vi "Working Thread.vi"(7 "EngineCSM":string, 10 "SocketName":string, 11 "Sequence":string) -> ()   [LabVIEW 2020, in "CSMStand(Lite).lvlib"]
uses:
  CSMStand(Lite).lvlib
  Typedef/Def-StepComplete Event Data.ctl
  162d78b0-f25f-4e28-9f32-62a227129c30.vi
  3235fbb5-1003-4f8d-8a8e-733f49405df1.vi
  29c90474-5633-4ebd-9475-c7049fde7730.vi
  07558781-58e1-4dd2-b95a-dcbf6018b6a4.vi
  <userlib>/_NEVSTOP/Communicable State Machine(CSM)/AdvanceAPI/CSM - Set Module Attribute.vi
  <userlib>/_NEVSTOP/Communicable State Machine(CSM)/addons/API-String-Arugments-Support/_Support/Data To API String Arguments.vi
  <userlib>/_NEVSTOP/Communicable State Machine(CSM)/AdvanceAPI/CSM - Get Module Attribute.vi
  <userlib>/_NEVSTOP/Communicable State Machine(CSM)/Communicable State Machine.lvlib
  <userlib>/_NEVSTOP/Communicable State Machine(CSM)/_Shared/CSM Shared.lvlib
  <userlib>/_NEVSTOP/Communicable State Machine(CSM)/addons/API-String-Arugments-Support/API String Arguments Support.lvlib
panel:
  in  "Debug Stop":bool
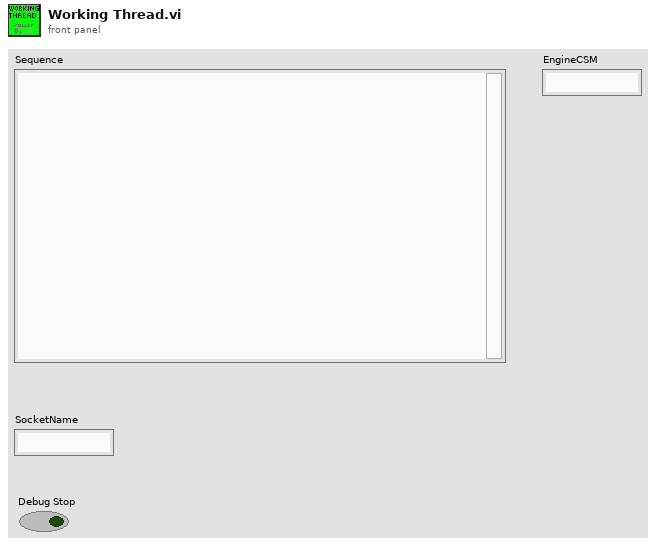
[diagram p1: front panel]
types:
  T1 = typedef "CSMStand(Lite).lvlib/Def-StepComplete Event Data.ctl" = cluster{"index":i32, "Arguments":string, "error":errorcluster}
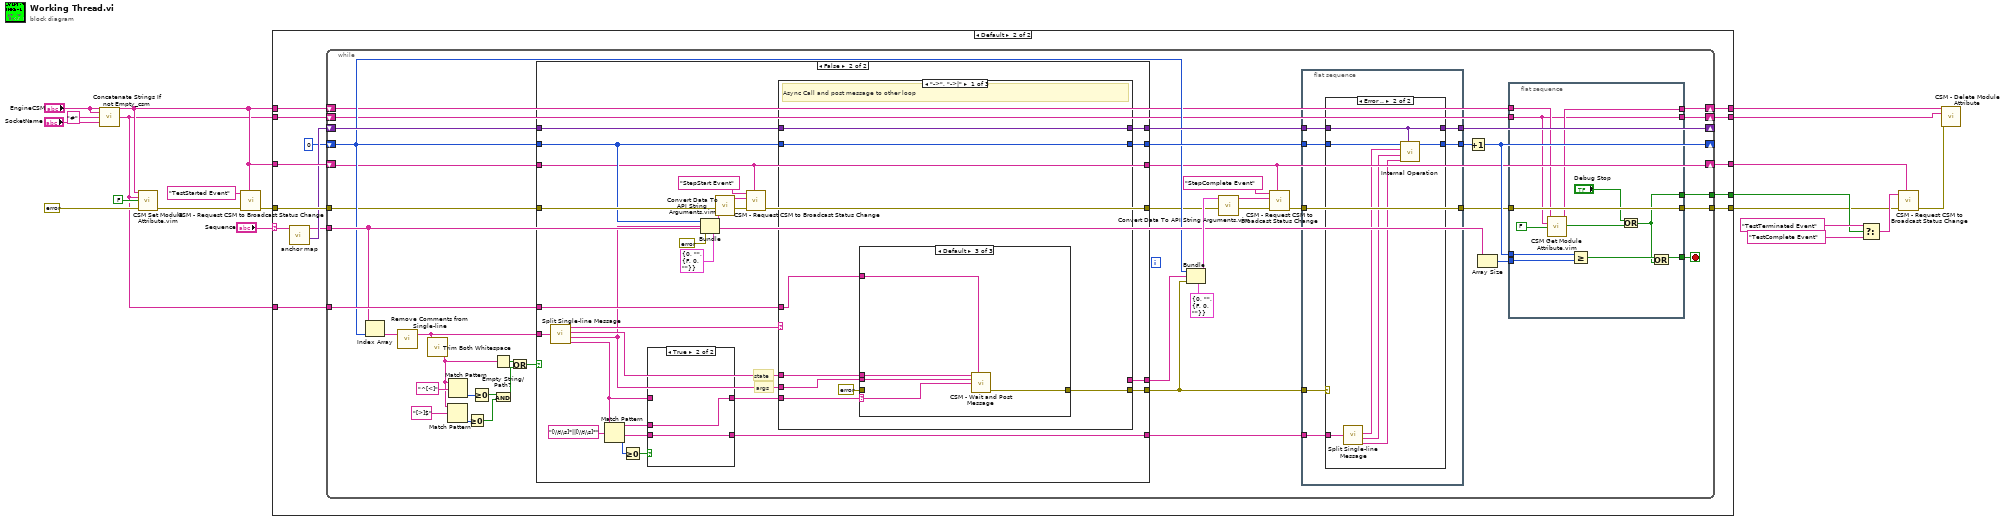
[diagram p0: block diagram]
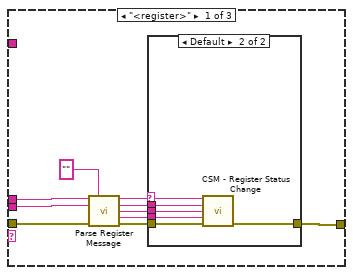
[diagram p6: hidden frame]
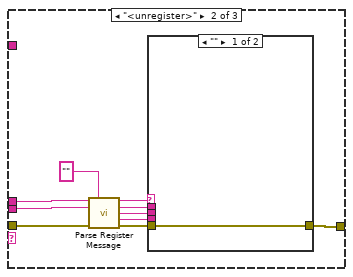
[diagram p8: hidden frame]
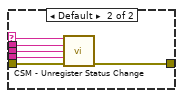
[diagram p9: hidden frame]
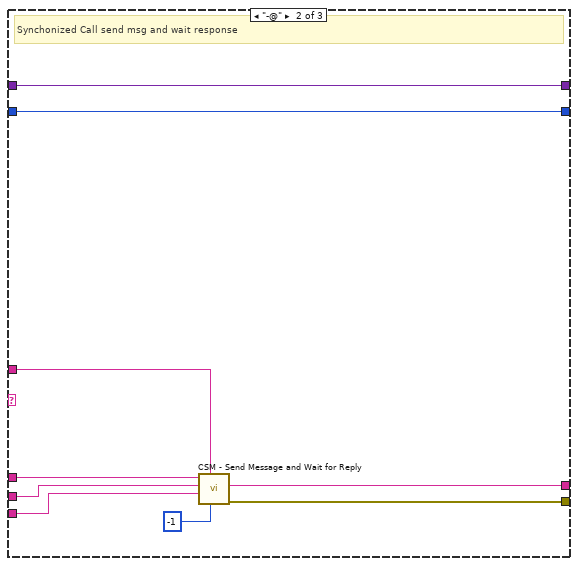
[diagram p10: hidden frame]
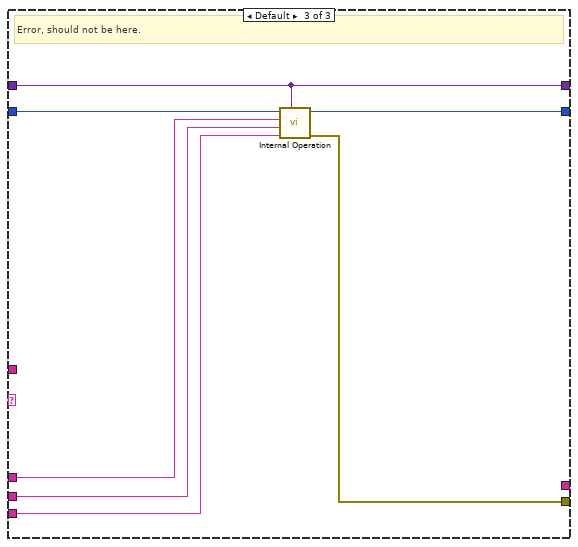
[diagram p11: hidden frame]
diagram:
  n1 = call <userlib>:"Concatenate Strings If not Empty_csm.vi"("String"="SocketName", "seperator(:)"="#", "prefix"="EngineCSM") -> ("result"=w1:string)  [unwired: 2 in]
  n2 = call "CSM Set Module Attribute.vim"("CSM Name"="EngineCSM", "Attribute"=w1, "Value"=FALSE, "Error In"=errorcluster {"status"=FALSE, "code"=0, "source"=""} ("error in (no error)")) -> ("error out"=w5:errorcluster)  [unwired: 8 in, 3 out]
  n3 = call <userlib>:"CSM - Request CSM to Broadcast Status Change.vi"("Module Name"="EngineCSM", "Error In (No Error)"=w5, "Status"="TestStarted Event") -> ("error out"=w18:errorcluster)  [unwired: 8 in]
  n4 = case shown="Default" "Sequence" {
    selector: "Sequence" -> [_ w31]
    tunnel: w18 -> [w22 w37]
    tunnel: "EngineCSM" -> [w23 w36]
    tunnel: [w23 w35] -> w17
    tunnel: [w22 w34] -> w9
    tunnel: w1 -> [_ w33]
    tunnel: "EngineCSM" -> [w21 w28]
    tunnel: [w21 w27] -> w12
    tunnel: [_ w26] -> w10
    tunnel: w1 -> [w20 w25]
    tunnel: [w20 w24] -> w6
    frame "False" {
    }
    frame Default {
      n5 = call "anchor map.vi"("string"=w31) -> ("Archt Map"=w32:variant, "Lines"=w30:string[])  [unwired: 9 in]
      n6 = while {
        tunnel: w37 -> [w43]
        tunnel: [w73] -> w34
        shift-right: [w40] -> w35
        shift-left: w36 -> [w41]
        tunnel: w33 -> [w80]
        tunnel: w30 -> [w70]
        shift-right: [w71] -> _
        shift-left: 0 -> [w47]
        shift-right: [w61] -> _
        shift-left: w32 -> [w68]
        shift-right: [w45] -> w27
        shift-left: w28 -> [w46]
        tunnel: [w44] -> w26
        shift-right: [w38] -> w24
        shift-left: w25 -> [w39]
        stop <- w74 stop-if-true
        n7 = Index Array(array=w70, index=w47) -> (element=w72:string)
        n8 = call <userlib>:"Remove Comments from Single-line.vi"("single-line text"=w72) -> ("single-line text without comments"=w52:string)  [unwired: 2 in]
        n9 = call <userlib>:"Trim Both Whitespace.vi"("String"=w52) -> ("Trimmed String"=w51:string)  [unwired: 1 in]
        n10 = Match Pattern(string=w51, regular expression="[>]$") -> (offset past match=w57:i32)  [unwired: 1 in, 3 out]
        n11 = Match Pattern(string=w51, regular expression="^[<]") -> (offset past match=w58:i32)  [unwired: 1 in, 3 out]
        n12 = Greater Or Equal To 0?(x=w57) -> (x >= 0?=w56:bool)
        n13 = Greater Or Equal To 0?(x=w58) -> (x >= 0?=w55:bool)
        n14 = Empty String/Path?(string/path=w51) -> (empty?=w53:bool)
        n15 = And(x=w55, y=w56) -> (x .and. y?=w54:bool)
        n16 = Or(x=w53, y=w54) -> (x .or. y?=w50:bool)
        n17 = case shown="False" w50 {
          tunnel: w80 -> [_ w138]
          tunnel: [_ w137] -> w64
          tunnel: [_ w136] -> w76
          tunnel: [w112 w135] -> w48
          tunnel: w47 -> [w112 w115]
          tunnel: w68 -> [w111 w134]
          tunnel: [_ w126] -> w63
          tunnel: [w111 w125] -> w62
          tunnel: w52 -> [_ w124]
          tunnel: w43 -> [w110 w120]
          tunnel: [w110 w119] -> w42
          tunnel: w41 -> [w109 w113]
          tunnel: [w109 w113] -> w40
          frame True {
          }
          frame False {
            # "args"
            # "state"
            n18 = call <userlib>:"Split Single-line Message.vi"("single-line text"=w124) -> ("operator"=w140:string, "state"=w139:string, "args"=w114:string, "source/target"=w129:string)  [unwired: 6 in]
            n19 = Match Pattern(string=w129, regular expression="[\\t\\s]*||[\\t\\s]*" ("string")) -> (before substring=w132:string, after substring=w127:string, offset past match=w131:i32)  [unwired: 1 in, 1 out]
            n20 = Greater Or Equal To 0?(x=w131) -> (x >= 0?=w130:bool)
            n21 = case shown="True" w130 {
              tunnel: w132 -> [_ w143]
              tunnel: w129 -> [w141 _]
              tunnel: [w141 w143] -> w128
              tunnel: w127 -> [_ w142]
              tunnel: [_ w142] -> w126
              frame False {
              }
              frame True {
              }
            }
            n22 = Bundle(cluster=T1 {"index"=0, "Arguments"="", "error"={"status"=FALSE, "code"=0, "source"=""}} ("output cluster"), "index"=w115, "Arguments"=w114, "error"=errorcluster {"status"=FALSE, "code"=0, "source"=""}) -> (w117:T1)
            n23 = call "Convert Data To API String Arguments.vim"("error in (no error)"=w120, "data"=w117) -> ("error out"=w122:errorcluster, "String"=w121:string)  [unwired: 6 in]
            n24 = call <userlib>:"CSM - Request CSM to Broadcast Status Change.vi"("Module Name"=w113, "Error In (No Error)"=w122, "Arguments (\"\")"=w121, "Status"="StepStart Event") -> ("error out"=w119:errorcluster)  [unwired: 7 in]
            n25 = case shown="\"->\", \"->|\"" w140 {
              tunnel: w139 -> [w147 w196 w201]
              tunnel: w114 -> [w146 w195 w200]
              tunnel: w138 -> [w148 w197 _]
              tunnel: w128 -> [w145 w194 w199]
              tunnel: [w149 w192 w202] -> w137
              tunnel: [_ w191 _] -> w136
              tunnel: [w151 w190 w204] -> w135
              tunnel: w115 -> [w151 w190 w203]
              tunnel: w134 -> [w150 w189 w198]
              tunnel: [w150 w189 w198] -> w125
              frame "->", "->|" {
                # "Async Call and post message to other loop"
                n26 = case shown="Default" w145 {
                  selector: w145 -> [_ _ w188]
                  tunnel: w146 -> [w155 w171 w187]
                  tunnel: w147 -> [w156 w172 w186]
                  tunnel: errorcluster {"status"=FALSE, "code"=0, "source"=""} ("error IO") -> [w154 w170 _]
                  tunnel: [w153 w169 w184] -> w149
                  tunnel: w148 -> [_ _ w185]
                  frame "<register>" {
                    n27 = call <userlib>:"Parse Register Message.vi"("State"=w156, "Module Name"="", "Args"=w155) -> ("Target"=w160:string, "Source"=w159:string, "Status"=w158:string, "Api"=w157:string)  [unwired: 8 in, 1 out]
                    n28 = case shown="Default" w160 {
                      selector: w160 -> [_ w167]
                      tunnel: w159 -> [_ w166]
                      tunnel: w158 -> [_ w165]
                      tunnel: w157 -> [_ w164]
                      tunnel: w154 -> [w161 w163]
                      tunnel: [w161 w162] -> w153
                      frame "" {
                      }
                      frame Default {
                        n29 = call <userlib>:"CSM - Register Status Change.vi"("CSM Name"=w167, "Source CSM Name (* as Default)"=w166, "Status"=w165, "Response Message (If \"\", Same as Source Message)"=w164, "Error In"=w163) -> ("error out"=w162:errorcluster)  [unwired: 9 in, 1 out]
                      }
                    }
                  }
                  frame "<unregister>" {
                    n30 = call <userlib>:"Parse Register Message.vi"("State"=w172, "Module Name"="", "Args"=w171) -> ("Target"=w176:string, "Source"=w175:string, "Status"=w174:string, "Api"=w173:string)  [unwired: 8 in, 1 out]
                    n31 = case shown="\"\"" w176 {
                      selector: w176 -> [_ w183]
                      tunnel: w175 -> [_ w182]
                      tunnel: w174 -> [_ w181]
                      tunnel: w173 -> [_ w180]
                      tunnel: w170 -> [w177 w179]
                      tunnel: [w177 w178] -> w169
                      frame "" {
                      }
                      frame Default {
                        n32 = call <userlib>:"CSM - Unregister Status Change.vi"("CSM Name"=w183, "Source CSM Name (* as Default)"=w182, "Status"=w181, "Response Message (\"*\" as Default)"=w180, "Error In"=w179) -> ("error out"=w178:errorcluster)  [unwired: 9 in, 1 out]
                      }
                    }
                  }
                  frame Default {
                    n33 = call <userlib>:"CSM - Wait and Post Message.vi"("State"=w186, "Current Module (\"\" to Generate an ID)"=w185, "Arguments (\"\")"=w187, "Target Module"=w188) -> ("error out"=w184:errorcluster)  [unwired: 11 in]
                  }
                }
              }
              frame "-@" {
                # "Synchonized Call send msg and wait response"
                n34 = call <userlib>:"CSM - Send Message and Wait for Reply.vi"("Response Timeout (-2 Using Global Settings)"=-1 ("Response Timeout(5000ms)"), "Current Module (\"\" to Generate an ID)"=w197, "Target Module"=w194, "Arguments (\"\")"=w195, "State"=w196) -> ("error out"=w192:errorcluster, "Response"=w191:string)  [unwired: 4 in, 1 out]
              }
              frame Default {
                # "Error, should not be here."
                n35 = call "Internal Operation.vi"("Archt Map"=w198, "source/target"=w199, "args"=w200, "state"=w201, "Numeric in"=w203) -> ("error out"=w202:errorcluster, "Numeric out"=w204:i32)  [unwired: 5 in]
              }
            }
          }
        }
        n36 = Bundle(cluster=T1 {"index"=0, "Arguments"="", "error"={"status"=FALSE, "code"=0, "source"=""}} ("output cluster"), "index"=w47, "Arguments"=w76, "error"=w64) -> (w75:T1)
        n37 = call "Convert Data To API String Arguments.vim"("error in (no error)"=w42, "data"=w75) -> ("error out"=w78:errorcluster, "String"=w77:string)  [unwired: 6 in]
        n38 = call <userlib>:"CSM - Request CSM to Broadcast Status Change.vi"("Module Name"=w40, "Error In (No Error)"=w78, "Arguments (\"\")"=w77, "Status"="StepComplete Event") -> ("error out"=w66:errorcluster)  [unwired: 7 in]
        n39 = flat-sequence {
          tunnel: [w85] -> w67
          tunnel: w48 -> [w84]
          tunnel: w66 -> [w87]
          tunnel: [w87] -> w65
          tunnel: w64 -> [w86]
          tunnel: w63 -> [w83]
          tunnel: w62 -> [w82]
          tunnel: [w81] -> w61
          frame #0 {
            n40 = case shown="Error .." w86 {
              tunnel: [w89 w95] -> w85
              tunnel: w84 -> [w89 w96]
              tunnel: w83 -> [_ w94]
              tunnel: w82 -> [w88 w90]
              tunnel: [w88 w90] -> w81
              frame No Error {
              }
              frame Error {
                n41 = call <userlib>:"Split Single-line Message.vi"("single-line text"=w94) -> ("state"=w93:string, "args"=w92:string, "source/target"=w91:string)  [unwired: 6 in, 1 out]
                n42 = call "Internal Operation.vi"("Archt Map"=w90, "source/target"=w91, "args"=w92, "state"=w93, "Numeric in"=w96) -> ("Numeric out"=w95:i32)  [unwired: 5 in, 1 out]
              }
            }
          }
        }
        n43 = Increment(x=w67) -> (x+1=w71:i32)
        n44 = Array Size(array=w70) -> (size(s)=w69:i32)
        n45 = flat-sequence {
          tunnel: [w108] -> w74
          tunnel: [w107] -> w73
          tunnel: w65 -> [w107]
          tunnel: w71 -> [w105]
          tunnel: w69 -> [w104]
          tunnel: w46 -> [w103]
          tunnel: [w102] -> w45
          tunnel: [w100] -> w44
          tunnel: w39 -> [w97]
          tunnel: [w97] -> w38
          frame #0 {
            n46 = call "CSM Get Module Attribute.vim"("CSM Name"=w103, "Attribute"=w97, "Default Value (Empty Variant)"=FALSE) -> ("CSM Name (Dup)"=w102:string, "Value"=w99:bool)  [unwired: 8 in, 3 out]
            n47 = Greater Or Equal?(x=w105, y=w104) -> (x >= y?=w106:bool)
            n48 = Or(x="Debug Stop", y=w99) -> (x .or. y?=w100:bool)
            n49 = Or(x=w106, y=w100) -> (x .or. y?=w108:bool)
          }
        }
      }
    }
  }
  n50 = Select(t="TestTerminated Event" ("Status"), s=w10, f="TestComplete Event" ("Status")) -> (s? t:f=w16:string)
  n51 = call <userlib>:"CSM - Request CSM to Broadcast Status Change.vi"("Module Name"=w17, "Error In (No Error)"=w9, "Status"=w16) -> ("error out"=w11:errorcluster)  [unwired: 8 in]
  n52 = call <userlib>:"CSM - Delete Module Attribute.vi"("CSM Name"=w12, "Attribute"=w6, "Error In"=w11) -> ()  [unwired: 9 in, 4 out]
